vi "System_Test_Create Dummy Objects.vi"() -> (3 "System.lvclass":refnum<class "System.lvclass">)   [LabVIEW 2015, in "System.lvclass"]
uses:
  System.lvclass
  AssetInterface/Interface_Asset.lvclass
  EnergyStorage/EnergyStorage.lvclass
  Grid/Grid.lvclass
  Load/Load.lvclass
  Dispatch Modules/SOC Control/Dispatch_SOC Control.lvclass
  Dispatch Modules/Demand Limiting/Dispatch_Demand Limiting.lvclass
  DispatchInterface/Interface_Dispatch.lvclass
  System.lvclass/System.ctl
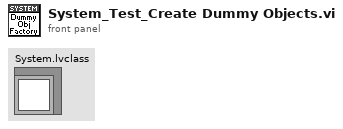
[diagram p1: front panel]
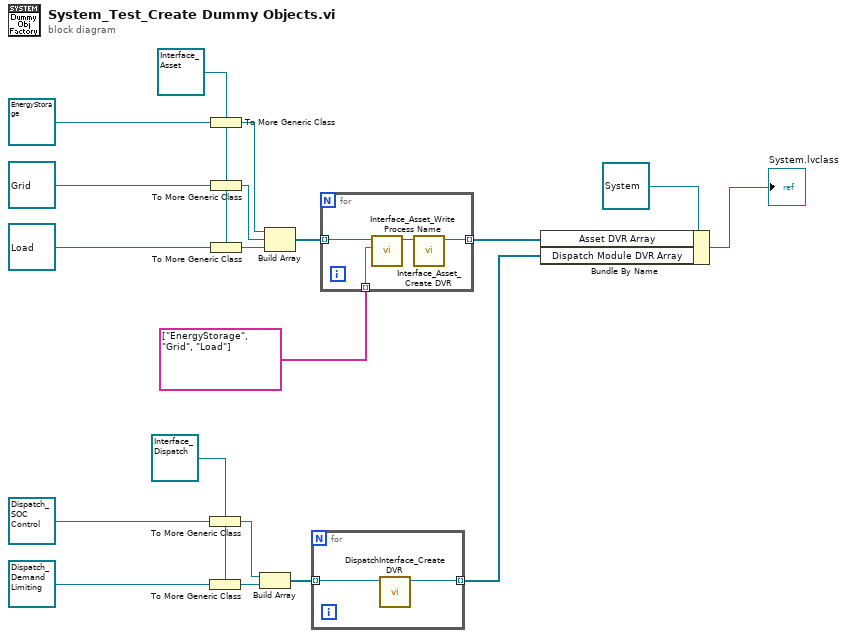
[diagram p0: block diagram]
diagram:
  w5 = refnum<class "Interface_Dispatch.lvclass"> refnum ("DispatchInterface.lvclass")
  w16 = refnum<class "Interface_Asset.lvclass"> refnum ("AssetInterface.lvclass")
  n1 = To More Generic Class(target class=w5, reference=refnum<class "Dispatch_SOC Control.lvclass"> refnum ("Dispatch_SOC Control.lvclass")) -> (generic class reference=w4:refnum<class "Interface_Dispatch.lvclass">)
  n2 = To More Generic Class(target class=w5, reference=refnum<class "Dispatch_Demand Limiting.lvclass"> refnum ("Dispatch_Demand Limiting.lvclass")) -> (generic class reference=w3:refnum<class "Interface_Dispatch.lvclass">)
  n3 = To More Generic Class(target class=w16, reference=refnum<class "EnergyStorage.lvclass"> refnum ("EnergyStorage.lvclass")) -> (generic class reference=w15:refnum<class "Interface_Asset.lvclass">)
  n4 = To More Generic Class(target class=w16, reference=refnum<class "Grid.lvclass"> refnum ("Grid.lvclass")) -> (generic class reference=w14:refnum<class "Interface_Asset.lvclass">)
  n5 = To More Generic Class(target class=w16, reference=refnum<class "Load.lvclass"> refnum ("Load.lvclass")) -> (generic class reference=w13:refnum<class "Interface_Asset.lvclass">)
  n6 = Build Array(w4, w3) -> (w2:refnum<class "Interface_Dispatch.lvclass">[])
  n7 = Build Array(w15, w14, w13) -> (w12:refnum<class "Interface_Asset.lvclass">[])
  n8 = for {
    tunnel: w2 -> [w21] mode=indexing
    tunnel: [w20] -> w1 mode=indexing
    n9 = call "DispatchInterface_Create DVR.vi"("DispatchInterface in"=w21) -> ("data value reference"=w20:refnum<data-value>)  [unwired: 9 in, 1 out]
  }
  n10 = for {
    tunnel: w12 -> [w25] mode=indexing
    tunnel: [w22] -> w8 mode=indexing
    tunnel: string[] ["EnergyStorage", "Grid", "Load"] -> [w24] mode=indexing
    n11 = call-dynamic "Interface_Asset_Write Process Name.vi"("Process Name"=w24, "AssetInterface in"=w25) -> ("AssetInterface out"=w23:refnum<class "Interface_Asset.lvclass">)  [unwired: 9 in]
    n12 = call "Interface_Asset_Create DVR.vi"("AssetInterface in"=w23) -> ("data value reference"=w22:refnum<data-value>)  [unwired: 9 in, 1 out]
  }
  n13 = Bundle By Name(cluster=refnum<class "System.lvclass"> refnum ("System.lvclass"), "Asset DVR Array"=w8, "Dispatch Module DVR Array"=w1) -> (→"System.lvclass":refnum<class "System.lvclass">)
